vi "Create_Trajectory_Read_Field_List.vi"() -> (0 "error out":errorcluster, 3 "section names":string[](array[string]))   [LabVIEW 2019]
uses:
  <vilib>/Utility/config.llb/NI_LVConfig.lvlib
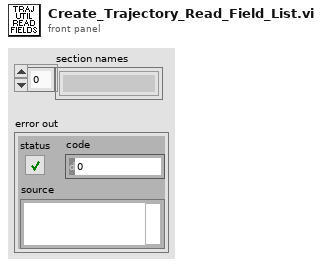
[diagram p1: front panel]
types:
  T1 = typedef "NI_LVConfig.lvlib/Config Data RefNum.ctl" = refnum<k1>
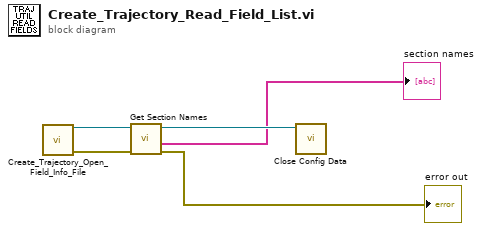
[diagram p0: block diagram]
diagram:
  n1 = call "Create_Trajectory_Open_Field_Info_File.vi"() -> ("error out"=w3:errorcluster, "Refnum out"=w1:T1)  [unwired: 10 in]
  n2 = call <vilib>:"Get Section Names.vi"("error in (no error)"=w3, "refnum"=w1) -> ("error out"=→"error out":errorcluster, "section names"=→"section names":string[], "refnum out"=w5:T1)  [unwired: 7 in]
  n3 = call <vilib>:"Close Config Data.vi"("refnum"=w5) -> ()  [unwired: 9 in, 2 out]
